vi "Send Single Trigger.vi"(8 "error in (no error)":errorcluster, 11 "VNA-Keysight PNA in":refnum<class "VNA-Keysight PNA.lvclass">) -> (0 "error out":errorcluster, 3 "VNA-Keysight PNA out":refnum<class "VNA-Keysight PNA.lvclass">)   [LabVIEW 2020, in "VNA-Keysight PNA.lvclass"]
doc: "Sent a single trigger for the VNA. It uses the OPC command to wait until completion.\nIt will use (sweeptime * N average * N ports) for the VISA timeout."
uses:
  VNA-Keysight PNA.lvclass
  C:/Sandbox/Git_Sandbox/WiSpry Test Framework source code (LV20)/WiSpry Test Framework/Instruments/Vector Network Analyzer/Vector Network Analyzer.lvclass
  C:/Sandbox/Git_Sandbox/WiSpry Test Framework source code (LV20)/WiSpry Test Framework/Instruments/Instrument.lvclass
  Instrument.lvclass/Instrument.ctl
  Vector Network Analyzer.lvclass/Vector Network Analyzer.ctl
  Instrument.lvclass
  <instrlib>/Keysight PNA Series/Keysight PNA Series.lvlib
  Vector Network Analyzer.lvclass
panel:
  out "Sweep Time":dbl
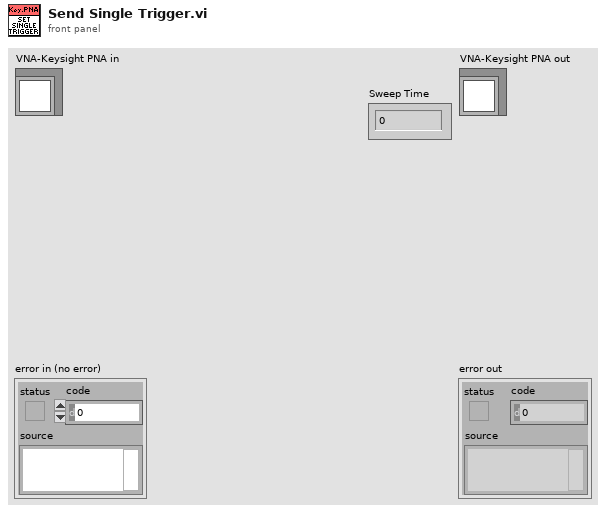
[diagram p1: front panel]
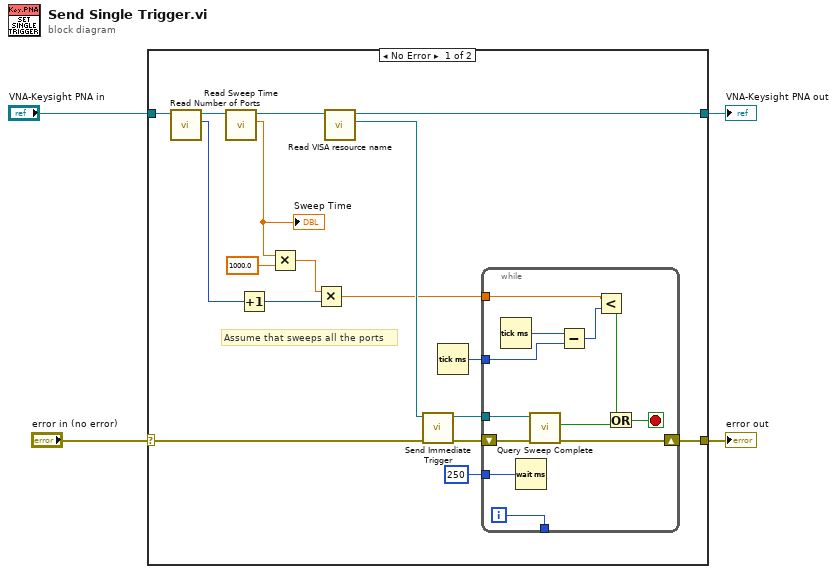
[diagram p0: block diagram]
diagram:
  n1 = case shown="No Error" "error in (no error)" {
    selector: "error in (no error)" -> [w20 w34]
    tunnel: [w21 w35] -> w3
    tunnel: "VNA-Keysight PNA in" -> [w8 w35]
    tunnel: [w17 w34] -> w1
    frame No Error {
      # "Assume that sweeps all the ports"
      n2 = call "Read Number of Ports.vi"("Vector Network Analyzer in"=w8) -> ("Number of Ports"=w6:i32, "Vector Network Analyzer out"=w7:refnum<class "VNA-Keysight PNA.lvclass">)  [unwired: 9 in]
      n3 = call "Read Sweep Time.vi"("Vector Network Analyzer in"=w7) -> ("Sweep Time"=w12:dbl, "Vector Network Analyzer out"=w14:refnum<class "VNA-Keysight PNA.lvclass">)  [unwired: 9 in]
      "Sweep Time" <- w12
      n4 = Increment(x=w6) -> (x+1=w5:i32)
      n5 = Multiply(x=w12, y=1000.0) -> (x*y=w10:dbl)
      n6 = Multiply(x=w10, y=w5) -> (x*y=w9:dbl)
      n7 = call "Read VISA resource name.vi"("Instrument in"=w14) -> ("VISA resource name"=w19:refnum<visa-resource-name>, "Instrument out"=w21:refnum<class "VNA-Keysight PNA.lvclass">)  [unwired: 9 in]
      n8 = call <instrlib>:"Send Immediate Trigger.vi"("error in (no error)"=w20, "VISA resource name"=w19) -> ("error out"=w18:errorcluster, "VISA resource name out"=w16:refnum<visa-resource-name>)  [unwired: 8 in]
      n9 = Tick Count (ms)() -> (millisecond timer value=w13:u32)
      n10 = while {
        tunnel: w16 -> [w31]
        shift-right: [w32] -> w17
        shift-left: w18 -> [w33]
        tunnel: u32 250 ("milliseconds to wait") -> [w30]
        tunnel: w13 -> [w29]
        tunnel: w9 -> [w25]
        tunnel: [w27] -> _
        i -> [w27]
        stop <- w22 stop-if-true
        n11 = Tick Count (ms)() -> (millisecond timer value=w28:u32)
        n12 = Wait (ms)(milliseconds to wait=w30) -> ()  [unwired: 1 out]
        n13 = call <instrlib>:"Query Sweep Complete.vi"("error in (no error)"=w33, "VISA resource name"=w31) -> ("error out"=w32:errorcluster, "Sweep Complete"=w26:bool)  [unwired: 7 in, 1 out]
        n14 = Subtract(x=w28, y=w29) -> (x-y=w24:u32)
        n15 = Less?(x=w25, y=w24) -> (x < y?=w23:bool)
        n16 = Or(x=w23, y=w26) -> (x .or. y?=w22:bool)
      }
    }
    frame Error {
    }
  }
  "error out" <- w1
  "VNA-Keysight PNA out" <- w3
